vi "SHAPE_decodeSet.vi"(3 "Parameters":i32[](array[numeric]), 5 "BandGlobalOpt.lvclass":refnum<class "Shapelets Search GA.lvclass">) -> (2 "Accuracy":sgl format="%.2f")   [LabVIEW 2016, in "Shapelets Search (GA).lvlib" / "Shapelets Search GA.lvclass"]
uses:
  Shapelets Search GA.lvclass
  Shapelets Search GA.lvclass/Shapelets Search GA.ctl
  <vilib>/Analysis/baseanly.llb/Normalize Vector.vi
  _Shapelets Search (Brute Force)/Shapelets Search (Brute Force).lvlib
  <vilib>/Analysis/NI_AALBase.lvlib
panel:
  # "This VI is a part of BCI Design library, http://www.ru-bci.org \nCopyright © 2020, Sotnikov Peter, All rights reserved. License: GNU GPLv3"
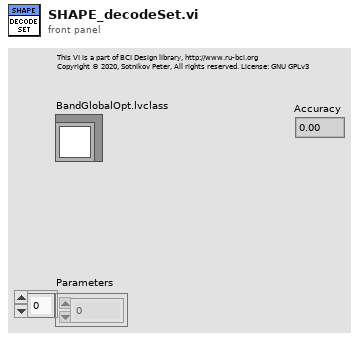
[diagram p1: front panel]
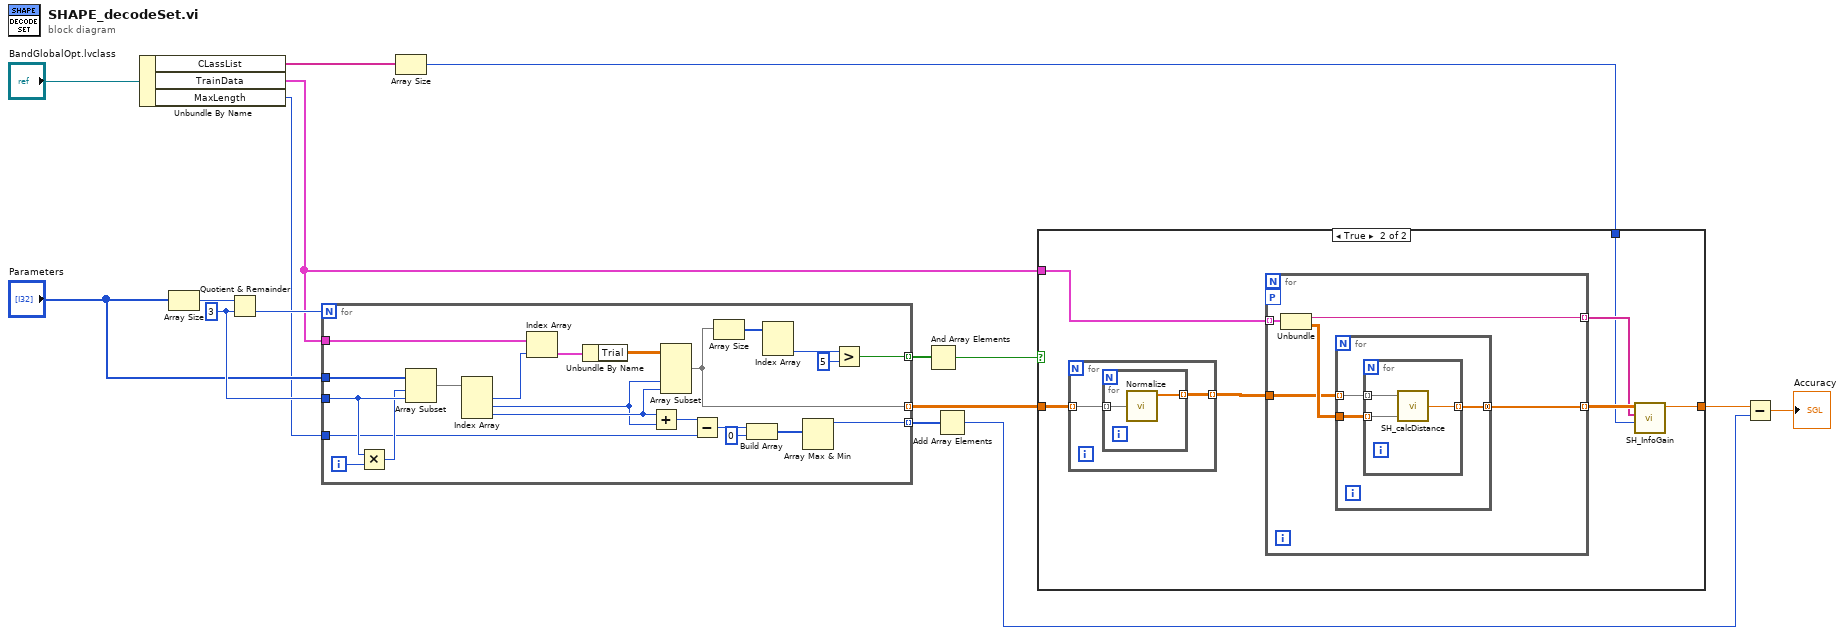
[diagram p0: block diagram]
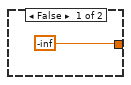
[diagram p2: hidden frame]
diagram:
  w12 = 3 ("y")
  n1 = Unbundle By Name("BandGlobalOpt.lvclass") -> ("CLassList"=w16:string[], "TrainData"=w9:cluster{"ClassLabel":string, "Trial":dbl[][]}[], "MaxLength"=w5:i32)
  n2 = Array Size(array="Parameters") -> (size(s)=w14:i32)
  n3 = Quotient & Remainder(x=w14, y=w12) -> (floor(x/y)=w13:i32)  [unwired: 1 out]
  n4 = for {
    N: w13 -> [_]
    tunnel: "Parameters" -> [w38]
    tunnel: w12 -> [w36]
    tunnel: w9 -> [w31]
    tunnel: [w26] -> w11 mode=indexing
    tunnel: [w25] -> w10 mode=indexing
    tunnel: w5 -> [w21]
    tunnel: [w17] -> w4 mode=indexing
    i -> [w37]
    n5 = Multiply(x=w36, y=w37) -> (x*y=w35:i32)
    n6 = Array Subset(array=w38, index=w35, length=w36) -> (w30:i32[])
    n7 = Index Array(array=w30) -> (element #1=w29:i32, element #2=w23:i32, element #3=w24:i32)  [unwired: 3 in]
    n8 = Index Array(array=w31, index=w29) -> (element=w34:cluster{"ClassLabel":string, "Trial":dbl[][]})
    n9 = Unbundle By Name(w34) -> ("Trial"=w33:dbl[][])
    n10 = Add(x=w24, y=w23) -> (x+y=w22:i32)
    n11 = Array Subset(array=w33, index (col)=w23, length (col)=w24) -> (w25:dbl[][])  [unwired: 2 in]
    n12 = Subtract(x=w22, y=w21) -> (x-y=w20:i32)
    n13 = Array Size(array=w25) -> (size(s)=w32:i32[])
    n14 = Build Array(w20, 0 ("element")) -> (w18:i32[])
    n15 = Index Array(array=w32) -> (element #2=w28:i32)  [unwired: 2 in, 1 out]
    n16 = Array Max & Min(array=w18) -> (max value=w17:i32)  [unwired: 3 out]
    n17 = Greater?(x=w28, y=5) -> (0:w26:bool)
  }
  n18 = Array Size(array=w16) -> (size(s)=w7:i32)
  n19 = And Array Elements(Boolean array=w11) -> (logical AND=w6:bool)
  n20 = Add Array Elements(numeric array=w4) -> (sum=w3:i32)
  n21 = case shown="True" w6 {
    tunnel: w10 -> [_ w46]
    tunnel: w9 -> [_ w45]
    tunnel: w7 -> [_ w41]
    tunnel: [-inf w40] -> w2
    frame False {
    }
    frame True {
      n22 = for {
        tunnel: w46 -> [w59] mode=indexing
        tunnel: [w58] -> w44 mode=indexing
        n23 = for {
          tunnel: [w61] -> w58 mode=indexing
          tunnel: w59 -> [w60] mode=indexing
          n24 = call-poly <vilib>:"Normalize.vi"("Vector"=w60) -> ("Normalized Vector"=w61:dbl[])  [unwired: 1 in, 3 out]
        }
      }
      n25 = for {
        tunnel: w45 -> [w51] mode=indexing
        tunnel: w44 -> [w49]
        workers-P: _ -> [_]
        tunnel: [w48] -> w42 mode=indexing
        tunnel: [w47] -> w43 mode=indexing
        n26 = Unbundle(w51) -> ("ClassLabel"=w48:string, "Trial"=w50:dbl[][])
        n27 = for {
          tunnel: w50 -> [w54]
          tunnel: w49 -> [w53] mode=indexing
          tunnel: [w52] -> w47 mode=concatenating
          n28 = for {
            tunnel: w54 -> [w56] mode=indexing
            tunnel: w53 -> [w57] mode=indexing
            tunnel: [w55] -> w52 mode=indexing
            n29 = call "SH_calcDistance.vi"("Time series"=w56, "Shapelet (normalized)"=w57) -> ("Distance out"=w55:dbl)  [unwired: 1 in]
          }
        }
      }
      n30 = call "SH_InfoGain.vi"("NumberOfClasses"=w41, "Class Labels"=w42, "Distancies"=w43) -> ("Accuracy"=w40:sgl)  [unwired: 7 in, 1 out]
    }
  }
  n31 = Subtract(x=w2, y=w3) -> (x-y=→"Accuracy":dbl)
